vi "Apply Symbols.vi"(8 "error in (no error)":errorcluster, 11 "Test Selector in":refnum<class "Test Selector.lvclass">) -> (0 "error out":errorcluster, 3 "Test Selector out":refnum<class "Test Selector.lvclass">)   [LabVIEW 2019, in "Test Selector.lvlib" / "Test Selector.lvclass"]
uses:
  Test Selector.lvclass
  Test Selector.lvclass/Test Selector.ctl
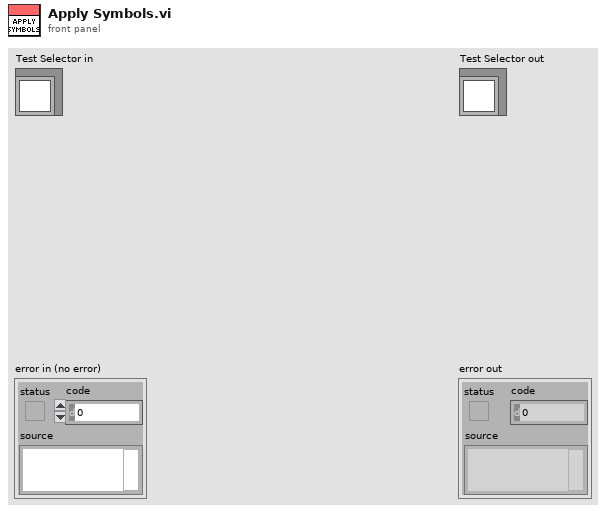
[diagram p1: front panel]
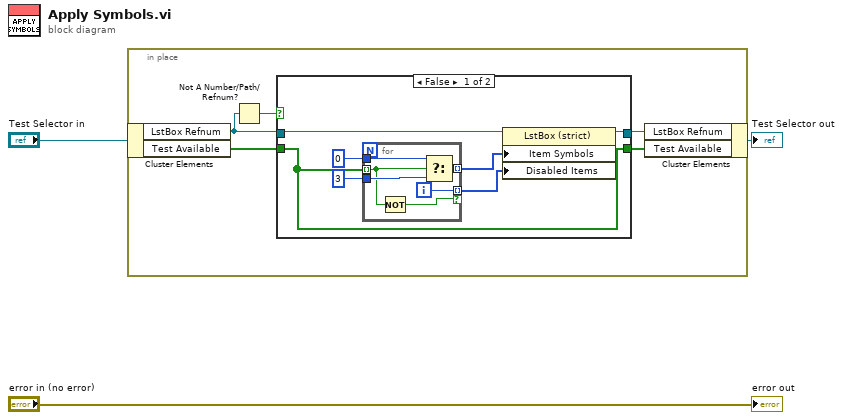
[diagram p0: block diagram]
diagram:
  n1 = in-place {
    n2 = in-place-cluster #1("Test Selector in") -> ("LstBox Refnum"=w7:refnum<vi>, "Test Available"=w5:bool[])
    n3 = Not A Number/Path/Refnum?(number/path/refnum=w7) -> (NaN/Path/Refnum?=w6:bool)
    n4 = case shown="False" w6 {
      tunnel: [w15 w23] -> w8
      tunnel: w7 -> [w14 w23]
      tunnel: w5 -> [w13 w22]
      tunnel: [w13 w22] -> w4
      frame False {
        n5 = for {
          tunnel: w13 -> [w18] mode=indexing
          tunnel: 0 -> [w21]
          tunnel: 3 -> [w19]
          tunnel: [w20] -> w10 mode=indexing
          tunnel: [w17] -> w9 mode=indexing if=w16
          i -> [w17]
          n6 = Not(x=w18) -> (.not. x?=w16:bool)
          n7 = Select(t=w21, s=w18, f=w19) -> (s? t:f=w20:i32)
        }
        n8 = property class="LstBox (strict)"(reference=w14, "Item Symbols"=w10, "Disabled Items"=w9) -> (reference out=w15:refnum<vi>)  [unwired: 1 in, 1 out]
      }
      frame True {
      }
    }
    n9 = in-place-cluster #1("LstBox Refnum"=w8, "Test Available"=w4) -> (→"Test Selector out":refnum<class "Test Selector.lvclass">)
  }
  "error out" <- "error in (no error)"
